vi "Max and min lift velocity.vi"() -> ()   [LabVIEW 2014]
panel:
  in  "Min Speed":dbl=0.7
  in  "Max Speed":dbl=1.0
  # "Min Speed needs to be pos because it is multiplyed neg joystick\nvalue (neg * neg would be positive :-)"
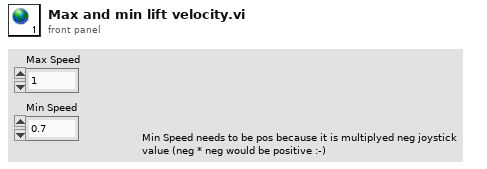
[diagram p1: front panel]
diagram:
